vi "open.local.publisher.file.vi"(8 "error in (no error)":errorcluster, 11 "publisher json":path) -> (0 "error out":errorcluster, 3 "publisher":T1)   [LabVIEW 2024, in "CV_Shared_Library.lvlib"]
uses:
  CV_Shared_Library.lvlib
  CV_RESTful_Library/typedefs/local_publisher--cluster.ctl
  <vilib>/addons/_JKI.lib/Serialization/JSON/JKI JSON Serialization.lvlib
  CV_RESTful_Library/CV_RESTful_Lib.lvlib
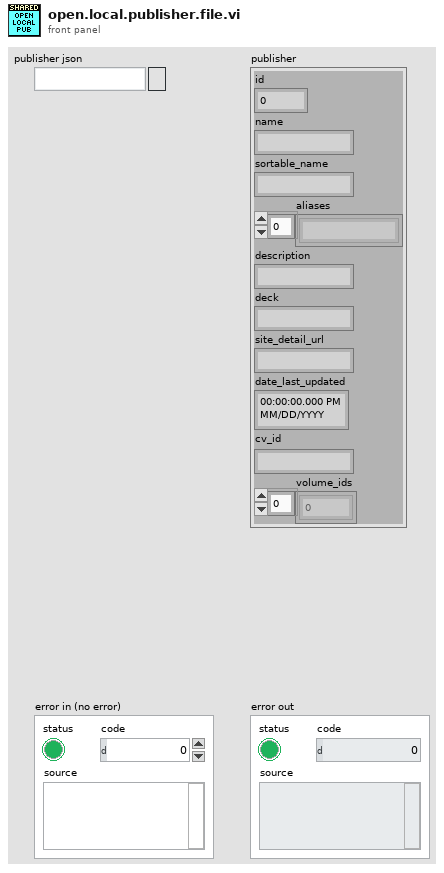
[diagram p1: front panel]
types:
  T1 = typedef "CV_RESTful_Lib.lvlib/local_publisher--cluster.ctl" = cluster{"id":i32, "name":string, "sortable_name":string, "aliases":string[], "description":string, "deck":string, "site_detail_url":string, "date_last_updated":timestamp, "cv_id":string, "volume_ids":i32[]}
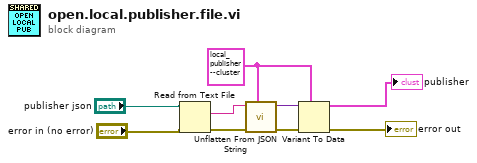
[diagram p0: block diagram]
diagram:
  w2 = T1 {"id"=0, "name"="", "sortable_name"="", "aliases"=[], "description"="", "deck"="", "site_detail_url"="", "date_last_updated"=timestamp(0 s since 1904-01-01), "cv_id"="", "volume_ids"=[]} ("publisher")
  n1 = Read from Text File(file (use dialog)="publisher json", error in="error in (no error)") -> (text=w4:string, error out=w5:errorcluster)  [unwired: 2 in, 2 out]
  n2 = call <vilib>:"Unflatten From JSON String.vi"("Type and Defaults"=w2, "error in"=w5, "JSON String"=w4) -> ("error out"=w6:errorcluster, "Variant"=w7:variant)  [unwired: 7 in]
  n3 = Variant To Data(error in=w6, type=w2, Variant=w7) -> (data=→"publisher":T1, error out=→"error out":errorcluster)
